vi "comet_thermo_get_values_MODBUS.vi"(8 "error in":errorcluster, 10 "Timeout":i32=5000, 11 "TCP ref in":refnum<k5>) -> (0 "error out":errorcluster, 1 "RH [%]":dbl, 2 "t [deg C]":dbl, 3 "TCP ref out":refnum<k5>, 4 "p [Pa]":dbl, 5 "p4":dbl)   [LabVIEW 2020]
uses:
  NI Modbus.llb/MB Modbus Command.ctl
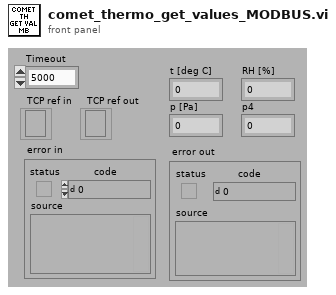
[diagram p1: front panel]
types:
  T1 = typedef "MB Modbus Command.ctl" = cluster{"Function Code":u8, "Starting Address":u16, "Quantity":u16, "Data":u16[], "Discrete":bool[]}
  T2 = cluster{"[0]":dbl, "[1]":dbl, "[2]":dbl, "[3]":dbl}
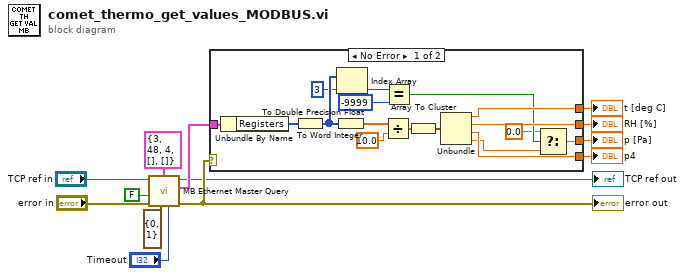
[diagram p0: block diagram]
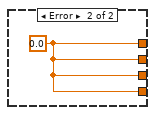
[diagram p2: hidden frame]
diagram:
  n1 = call "MB Ethernet Master Query.vi"("Timeout"="Timeout", "MBAP Header"=cluster{"Transaction ID":u16, "Unit ID":u8} {"Transaction ID"=0, "Unit ID"=1}, "error in (no error)"="error in", "Use MODBUS Data Unit?"=FALSE, "Modbus Command"=T1 {"Function Code"=3, "Starting Address"=48, "Quantity"=4, "Data"=[], "Discrete"=[]}, "TCP Connection Refnum in"="TCP ref in") -> ("error out"=w7:errorcluster, "Registers"=w9:cluster{"Registers":u16[], "Discrete":bool[]}, "TCP Connection Refnum (dup)"=→"TCP ref out":refnum<k5>)  [unwired: 1 in, 2 out]
  "error out" <- w7
  n2 = case shown="No Error" w7 {
    tunnel: w9 -> [w30 _]
    tunnel: [w26 w31] -> w4
    tunnel: [w25 w31] -> w3
    tunnel: [w20 w31] -> w2
    tunnel: [w24 w31] -> w1
    frame No Error {
      n3 = Unbundle By Name(w30) -> ("Registers"=w29:u16[])
      n4 = To Word Integer(number=w29) -> (16bit integer=w21:i16[])
      n5 = To Double Precision Float(number=w21) -> (double precision float=w23:dbl[])
      n6 = Index Array(array=w21, index=3) -> (element=w19:i16)
      n7 = Divide(x=w23, y=10.0) -> (x/y=w22:dbl[])
      n8 = Equal?(x=w19, y=i16 -9999) -> (x = y?=w17:bool)
      n9 = Array To Cluster(array=w22) -> (cluster=w27:T2)
      n10 = Unbundle(w27) -> ("[0]"=w26:dbl, "[1]"=w25:dbl, "[2]"=w24:dbl, "[3]"=w16:dbl)
      n11 = Select(t=0.0, s=w17, f=w16) -> (s? t:f=w20:dbl)
    }
    frame Error {
      w31 = 0.0 ("[0]")
    }
  }
  "t [deg C]" <- w4
  "RH [%]" <- w3
  "p [Pa]" <- w2
  "p4" <- w1
